vi "Module Identities.vi"(8 "error in (no error)":errorcluster, 11 "GUI Helper in":refnum<class "GUI Helper.lvclass">) -> (0 "error out":errorcluster, 2 "Identities":refnum<class "Identity.lvclass">[](array[class]), 3 "GUI Helper out":refnum<class "GUI Helper.lvclass">)   [LabVIEW 2020, in "VolatusGUI.lvlib" / "GUI Helper.lvclass"]
uses:
  GUI Helper.lvclass
  Volatus/Identity/Identity.lvclass
  GUI Helper.lvclass/GUI Helper.ctl
  GUI Identity/GUI Identity.lvclass
  C:/dev/lv20CE/relink/lv-volatus/Volatus/Identity/Identity.lvclass
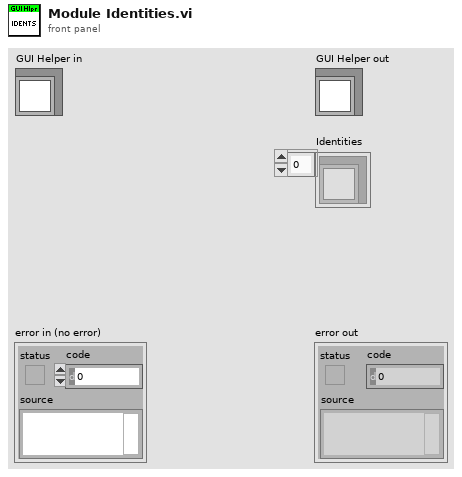
[diagram p1: front panel]
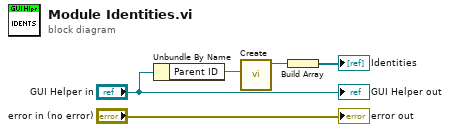
[diagram p0: block diagram]
diagram:
  n1 = Unbundle By Name("GUI Helper in") -> ("Parent ID"=w1:string)
  n2 = call "Create.vi"("Module ID"=w1) -> ("GUI Identity out"=w4:refnum<class "GUI Identity.lvclass">)  [unwired: 10 in]
  n3 = Build Array(w4) -> (→"Identities":refnum<class "GUI Identity.lvclass">[])
  "error out" <- "error in (no error)"
  "GUI Helper out" <- "GUI Helper in"
